vi "Read From File.vi"(8 "error in (no error)":errorcluster, 11 "file path":path) -> (0 "error out":errorcluster, 2 "input cfg JSON":string, 3 "input type":T1 caption="master clock source", 5 "file exists?":bool)   [LabVIEW 2022 SP3, in "input cfg file.lvlib"]
uses:
  input cfg file.lvlib
  controls/input type.ctl
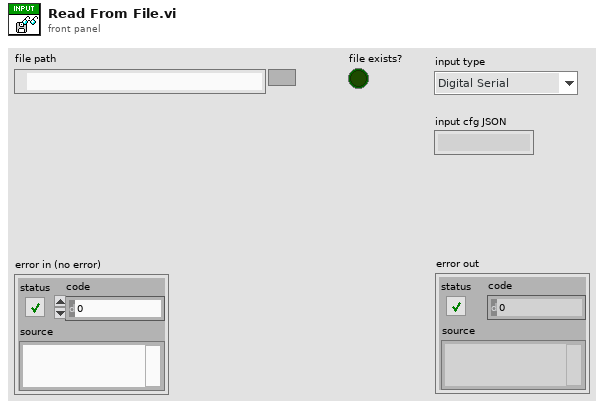
[diagram p1: front panel]
types:
  T1 = typedef "input type.ctl" = enum32{"Digital Serial", "PDM"}
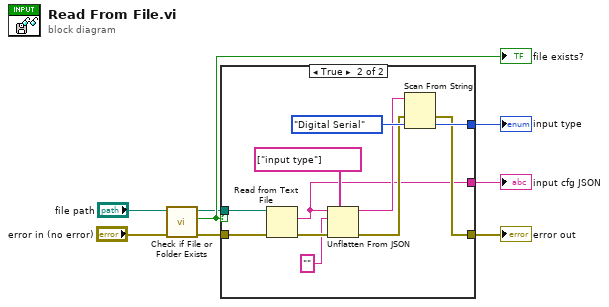
[diagram p0: block diagram]
diagram:
  n1 = call <vilib>:"Check if File or Folder Exists.vi"("error in (no error)"="error in (no error)", "path"="file path") -> ("error out"=w7:errorcluster, "file or folder exists?"=w6:bool, "dup path"=w5:path)  [unwired: 7 in]
  "file exists?" <- w6
  n2 = case shown="True" w6 {
    tunnel: w7 -> [w9 w19]
    tunnel: w5 -> [_ w20]
    tunnel: [w9 w11] -> w3
    tunnel: [_ w13] -> w2
    tunnel: [_ w10] -> w1
    frame False {
      # "no file found"
    }
    frame True {
      n3 = Read from Text File(file (use dialog)=w20, error in=w19) -> (text=w10:string, error out=w18:errorcluster)  [unwired: 2 in, 2 out]
      n4 = Unflatten From JSON(path=string[] ["input type"], JSON string=w10, type and defaults="", error in (no error)=w18) -> (value=w14:string, error out=w12:errorcluster)  [unwired: 3 in]
      n5 = Scan From String(input string=w14, error in=w12, default 1=input_type."Digital Serial" ("input type")) -> (error out=w11:errorcluster, output 1=w13:T1)  [unwired: 2 in, 2 out]
    }
  }
  "error out" <- w3
  "input type" <- w2
  "input cfg JSON" <- w1
